vi "Pump_stage.vi"(0 "Start":bool, 1 "N_pump_on":u32, 2 "N_pump_on_ref":u32, 3 "Num_pump_on_ref":u32, 4 "N_pump":u32, 7 "T_pump_on_time":u32, 9 "N_pump_on_ref_alr":bool) -> (14 "N curr":u32, 15 "+1":bool, 16 "ok":bool, 17 "not ok":bool, 18 "t":u32)   [LabVIEW 2019]
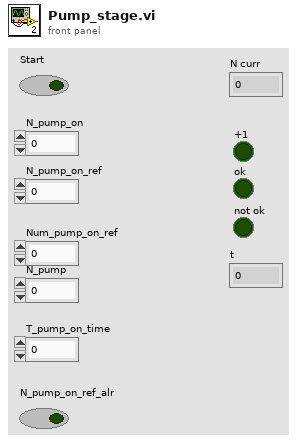
[diagram p1: front panel]
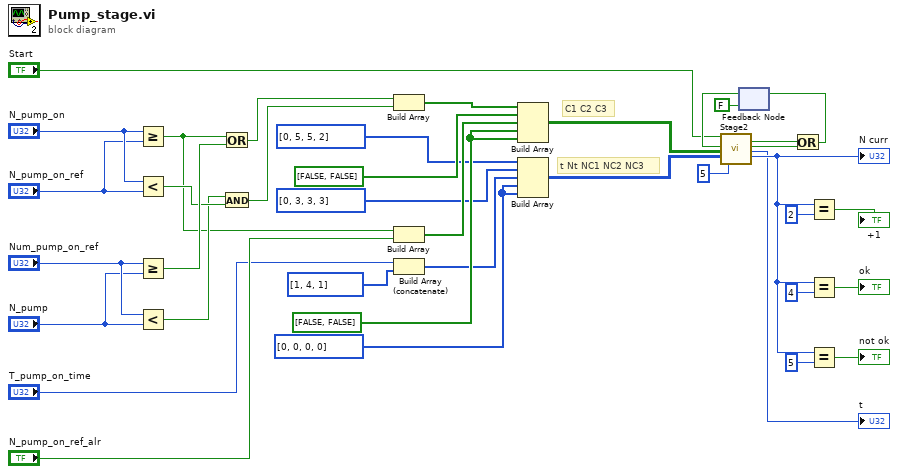
[diagram p0: block diagram]
diagram:
  w11 = u32[] [0, 0, 0, 0] ("Stage table")
  w10 = bool[] [FALSE, FALSE]
  # "C1 C2 C3"
  # "t Nt NC1 NC2 NC3"
  n1 = Greater Or Equal?(x="N_pump_on", y="N_pump_on_ref") -> (x >= y?=w24:bool)
  n2 = Less?(x="N_pump_on", y="N_pump_on_ref") -> (x < y?=w33:bool)
  n3 = Greater Or Equal?(x="Num_pump_on_ref", y="N_pump") -> (x >= y?=w34:bool)
  n4 = Less?(x="Num_pump_on_ref", y="N_pump") -> (x < y?=w32:bool)
  n5 = Or(x=w24, y=w34) -> (x .or. y?=w2:bool)
  n6 = And(x=w32, y=w33) -> (x .and. y?=w27:bool)
  n7 = Build Array(w2, w27) -> (w5:bool[])
  n8 = Build Array(w24, "N_pump_on_ref_alr") -> (w8:bool[])
  n9 = Build Array (concatenate)("T_pump_on_time", u32[] [1, 4, 1] ("Stage table")) -> (w9:u32[])
  n10 = Build Array(w5, bool[] [FALSE, FALSE], w8, w10, w10) -> (w26:bool[][])
  n11 = Build Array(u32[] [0, 5, 5, 2] ("Stage table"), u32[] [0, 3, 3, 3] ("Stage table"), w9, w11, w11) -> (w20:u32[][])
  n12 = feedback #1(FALSE) -> (w35:bool)
  n13 = call "Stage2.vi"("Start"="Start", "Reset"=w35, "C"=w26, "Stage table"=w20, "End step"=u32 5) -> ("Stop"=w38:bool, "End"=w37:bool, "t"=→"t":u32, "N curr"=w19:u32)  [unwired: 9 in, 2 out]
  "N curr" <- w19
  n14 = Or(x=w38, y=w37) -> (x .or. y?=w36:bool)
  n15 = feedback-in #1(w36) -> ()
  n16 = Equal?(x=w19, y=u32 2) -> (x = y?=→"+1":bool)
  n17 = Equal?(x=w19, y=u32 4) -> (x = y?=→"ok":bool)
  n18 = Equal?(x=w19, y=u32 5) -> (x = y?=→"not ok":bool)
